vi "temp_monitor.vi"() -> ()   [LabVIEW 2013]
uses:
  <vilib>/Platform/TimedLoop/XDataNode/timing_clust.ctl
  <vilib>/Platform/TimedLoop/XDataNode/nitl_modes.ctl
  <vilib>/Platform/TimedLoop/XDataNode/wakeup.ctl
  <vilib>/platform/TimedLoop/XDataNode/XDataNode.xnode
  <vilib>/Platform/TimedLoop/XDataNode/XDNodeRunTimeDep.lvlib
panel:
  in  "Measurement Period (ms)":i64=10000
  in  "stop":bool
  out "Temp":dbl=26.64 format="%.2g"
  out "Temperature vs. Time":waveform(dbl)(graph)={"t0"=timestamp(3450374135.2304688 s since 1904-01-01), "dt"=1.0, "Y"=[26.64]}
  in  "COM Port":u16=4
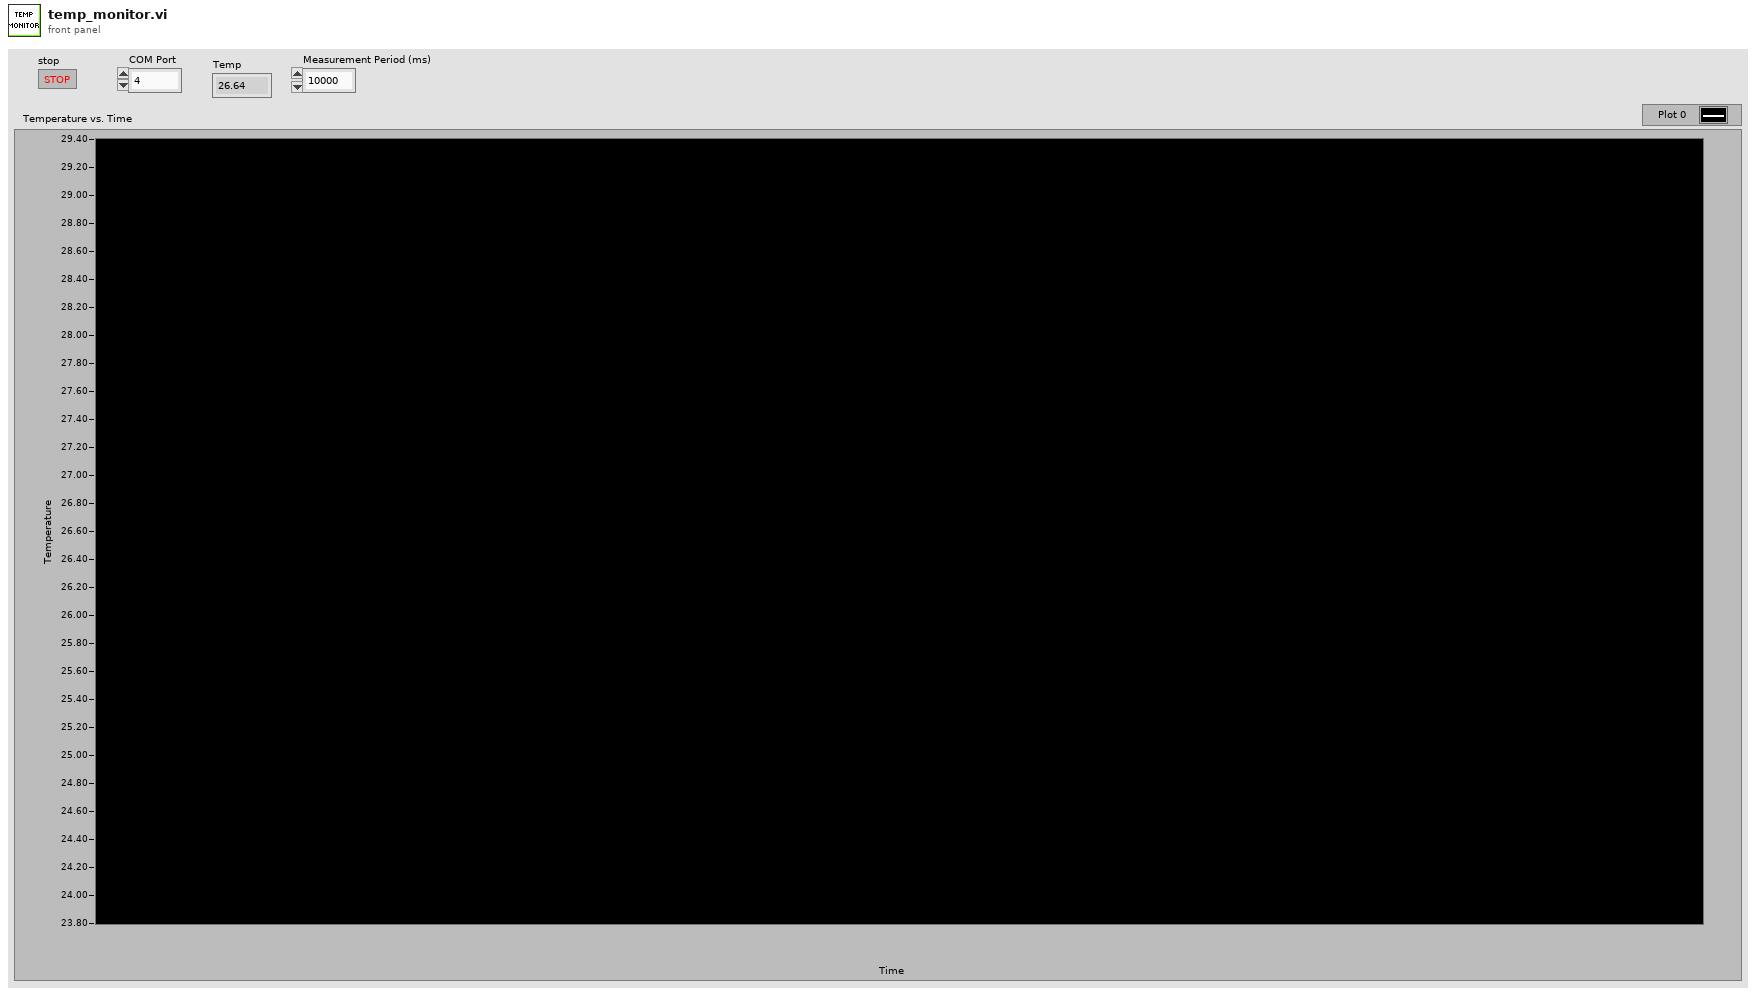
[diagram p1: front panel]
types:
  T1 = typedef "XDNodeRunTimeDep.lvlib/timing_clust.ctl" = cluster{"Expected End [f-1]":u64, "Actual End [f-1]":u64, "Finished Late? [f-1]":bool, "Expected End [i-1]":u64, "Actual End [i-1]":u64, "Finished Late? [i-1]":bool, "Expected Start [i]":u64, "Actual Start [i]":u64, "Expected Start [f]":u64, "Actual Start [f]":u64, "Source Name":string, "Structure Name":string, "Period":i64, "Deadline":i64, "Offset":i64, "Start":i64, "Priority":i32, "Timeout":i32, "Mode":T2, "Wakeup Reason":T3, "Error":errorcluster, "Source Type":string, "Secondary Source Type":string, "Global End Time":u64, "Global Start Time":u64, "Frame Duration":u64, "Iteration Duration":u64, "Assigned CPU":i32, "I/O Scan Engine Mode":u32}
  T2 = typedef "XDNodeRunTimeDep.lvlib/nitl_modes.ctl" = enum32{"No Change", "Process missed periods, maintain original phase", "Discard missed periods, maintain original phase", "Process missed periods, ignore original phase", "Discard missed periods, ignore original phase"}
  T3 = typedef "XDNodeRunTimeDep.lvlib/wakeup.ctl" = enum32{"Normal", "Aborted", "Asynchronous wakeup", "Timing source error", "Timed loop error", "Timeout"}
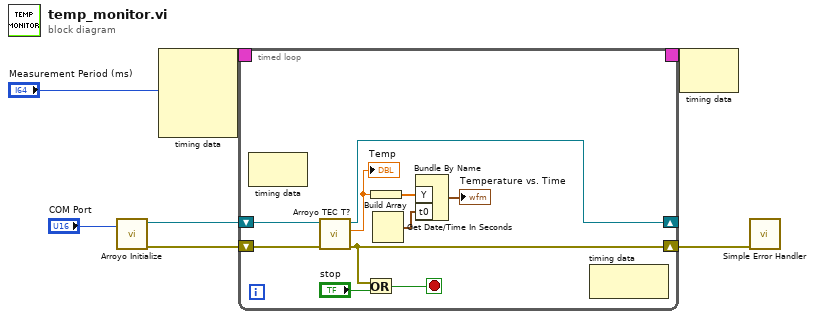
[diagram p0: block diagram]
diagram:
  n1 = call "Arroyo Initialize.vi"("COM Port"="COM Port") -> ("dup VISA resource name"=w6:refnum<visa-resource-name>, "error out"=w4:errorcluster)  [unwired: 3 in]
  n2 = node-c288("Measurement Period (ms)") -> (w3:T1)  [unwired: 3 in]
  n3 = timed-loop {
    shift-right: [w14] -> w5
    shift-left: w4 -> [w16]
    shift-right: [w15] -> _
    shift-left: w6 -> [w17]
    timing: w3 -> [_]
    timing-out: [_] -> w2
    stop <- w12 stop-if-true
    n4 = node-c288() -> ()  [unwired: 1 in, 1 out]
    n5 = call "Arroyo TEC T?.vi"("error in (no error)"=w16, "VISA resource name"=w17) -> ("error out"=w14:errorcluster, "TEC Temperature"=w11:dbl, "dup VISA resource name"=w15:refnum<visa-resource-name>)  [unwired: 3 in]
    "Temp" <- w11
    n6 = Or(x=w14, y="stop") -> (x .or. y?=w12:bool)
    n7 = Build Array(w11) -> (w10:dbl[])
    n8 = Get Date/Time In Seconds() -> (seconds since 1Jan1904=w9:timestamp)
    n9 = Bundle By Name("Y"=w10, "t0"=w9) -> (→"Temperature vs. Time":waveform(dbl))  [unwired: 1 in]
    n10 = node-c288() -> ()  [unwired: 1 in, 1 out]
  }
  n11 = node-c288(w2) -> ()  [unwired: 1 out]
  n12 = call <vilib>:"Simple Error Handler.vi"("error in (no error)"=w5) -> ()  [unwired: 4 in, 5 out]
